vi "RSZVB Set Restart Behavior.vi"(8 "error in (no error)":errorcluster {"code" format="%.0x"}, 9 "Restart Behavior (Set All Traces To Zero)":i32(ring)=1 items=["Keep Previous Measurement", "Set All Traces To Zero"], 11 "VISA session":refnum<visa-resource-name>) -> (0 "error out":errorcluster {"code" format="%.0x"}, 3 "dup VISA session":refnum<visa-resource-name>)   [LabVIEW 2011]
doc: "This VI Defines the restart behavior of the instrument.\n\nRemote-control command(s):\nSYSTem:TRESet[:STATe] <Boolean>"
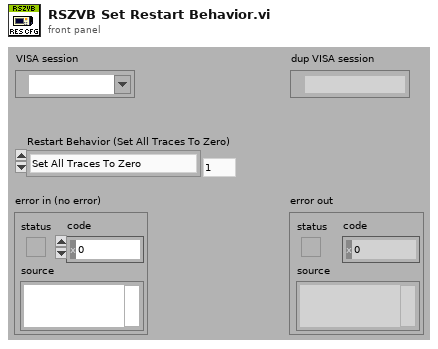
[diagram p1: front panel]
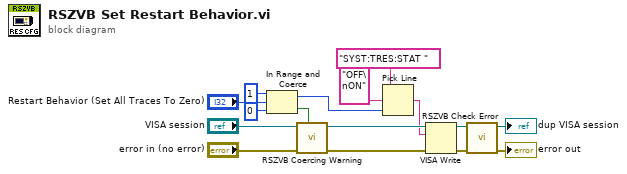
[diagram p0: block diagram]
diagram:
  n1 = In Range and Coerce(upper limit=1, x="Restart Behavior (Set All Traces To Zero)", lower limit=0) -> (coerced(x)=w3:i32, In Range?=w6:bool)
  n2 = call "RSZVB Coercing Warning.vi"("In Range?"=w6, "error in (no error)"="error in (no error)", "VISA session"="VISA session") -> ("error out"=w15:errorcluster, "dup VISA session"=w16:refnum<visa-resource-name>)  [unwired: 7 in]
  n3 = Pick Line(string ("")="SYST:TRES:STAT ", multi-line string="OFF\nON", line index=w3) -> (output string=w1:string)
  n4 = VISA Write(VISA resource name=w16, write buffer=w1, error in (no error)=w15) -> (VISA resource name out=w13:refnum<visa-resource-name>, error out=w14:errorcluster)  [unwired: 1 out]
  n5 = call "RSZVB Check Error.vi"("error in (no error)"=w14, "VISA session"=w13) -> ("error out"=→"error out":errorcluster, "dup VISA session"=→"dup VISA session":refnum<visa-resource-name>)  [unwired: 8 in]
